vi "buildWithCLI.vi"   [LabVIEW 2019]
uses:
  <vilib>/Wiresmith Technology/G CLI/CLI Class/CLI.lvclass
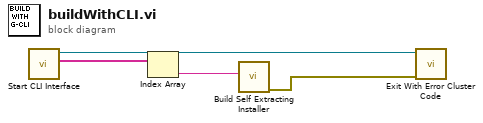
[diagram p0: block diagram]
diagram:
  n1 = call <vilib>:"Start CLI Interface.vi"() -> ("Custom Parameters"=w3:string[], "CLI out"=w2:refnum<class "CLI.lvclass">)  [unwired: 8 in, 2 out]
  n2 = Index Array(array=w3) -> (element=w4:string)  [unwired: 1 in]
  n3 = call "Build Self Extracting Installer.vi"("Package Version"=w4) -> ("Error Out"=w1:errorcluster)  [unwired: 10 in]
  n4 = call <vilib>:"Exit With Error Cluster Code.vi"("error in (no error)"=w1, "CLI in"=w2) -> ()  [unwired: 9 in, 1 out]
